vi "Discrete Transfer Function (DBL).vi"(2 "initialize":bool, 3 "transfer function":cluster{"numerator":dbl[], "denominator":dbl[]} {"denominator" format="%.2f"; "numerator" format="%.2f"}, 5 "input point":dbl format="%.2f") -> (1 "output point":dbl format="%.2f")   [LabVIEW 2020, in "NI_AdvCtrl_discrete linear.lvlib"]
doc: "LabVIEW no longer supports this VI. You can obtain similar functionality by installing the LabVIEW Simulation Module.\n\nCalculates the new output point, where the transfer function and the input point are given. The transfer function is described by two polynomials, numerator and denominator."
uses:
  <vilib>/addons/control/advanced/NI_AdvCtrl_discrete linear.lvlib
  <vilib>/addons/control/advanced/NI_AdvCtrl_continuous linear.lvlib
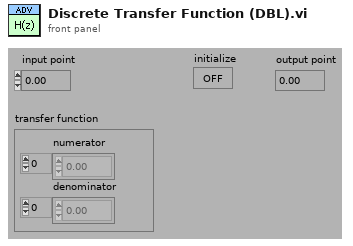
[diagram p1: front panel]
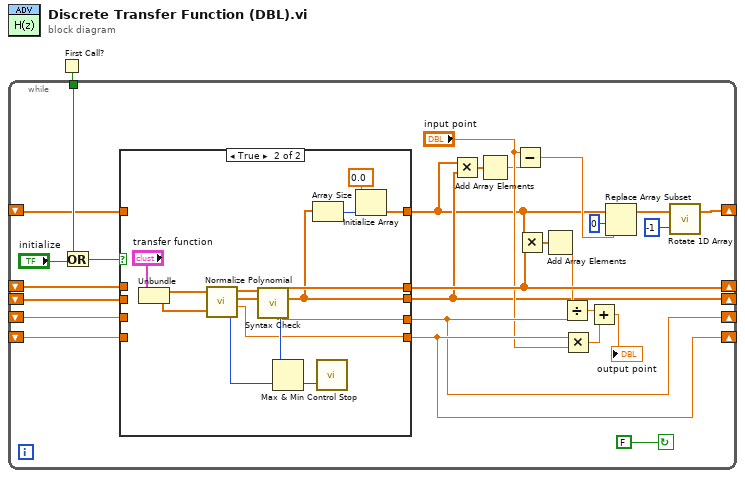
[diagram p0: block diagram]
diagram:
  n1 = First Call?() -> (First Call?: T/F=w1:bool)
  n2 = while {
    shift-left: _ -> [w13]
    shift-right: [w3] -> _
    tunnel: w1 -> [w17]
    shift-left: _ -> [w23]
    shift-right: [w22] -> _
    shift-left: _ -> [w24]
    shift-right: [w21] -> _
    shift-left: _ -> [w25]
    shift-right: [w7] -> _
    shift-left: _ -> [w26]
    shift-right: [w12] -> _
    stop <- FALSE continue-if-true
    n3 = Or(x=w17, y="initialize") -> (x .or. y?=w16:bool)
    n4 = case shown="True" w16 {
      tunnel: [w30 w44] -> w22
      tunnel: [w31 w43] -> w21
      tunnel: [w33 w42] -> w12
      tunnel: [w32 w39] -> w7
      tunnel: w26 -> [w33 _]
      tunnel: w25 -> [w32 _]
      tunnel: w24 -> [w31 _]
      tunnel: w23 -> [w30 _]
      tunnel: [w29 w38] -> w6
      tunnel: w13 -> [w29 _]
      frame False {
      }
      frame True {
        n5 = Unbundle("transfer function") -> ("numerator"=w37:dbl[], "denominator"=w36:dbl[])
        n6 = call <vilib>:"Normalize Polynomial.vi"("Numerator"=w37, "Denominator"=w36) -> ("Numerator new"=w45:dbl[], "Denominator new"=w46:dbl[], "additive constant"=w44:dbl, "error"=w47:i32)
        n7 = call <vilib>:"Syntax Check.vi"("Denominator"=w46, "Numerator"=w45) -> ("error"=w48:i32, "gain"=w43:dbl, "Denominator new"=w39:dbl[], "Numerator new"=w42:dbl[])  [unwired: 1 out]
        n8 = Max & Min(x=w48, y=w47) -> (min(x,y)=w35:i32)  [unwired: 1 out]
        n9 = Array Size(array=w39) -> (size(s)=w40:i32)
        n10 = call <vilib>:"Control Stop.vi"("error"=w35) -> ()  [unwired: 2 out]
        n11 = Initialize Array(0.0, w40) -> (w38:dbl[])
      }
    }
    n12 = Multiply(x=w6, y=w7) -> (x*y=w8:dbl[])
    n13 = Add Array Elements(numeric array=w8) -> (sum=w5:dbl)
    n14 = Subtract(x="input point", y=w5) -> (x-y=w15:dbl)
    n15 = Multiply(x=w6, y=w12) -> (x*y=w11:dbl[])
    n16 = Add Array Elements(numeric array=w11) -> (sum=w10:dbl)
    n17 = Divide(x=w10, y=w21) -> (x/y=w27:dbl)
    n18 = Multiply(x=w22, y="input point") -> (x*y=w28:dbl)
    n19 = Add(x=w27, y=w28) -> (x+y=→"output point":dbl)
    n20 = Replace Array Subset(array=w6, new element=w15, index=0 ("Index")) -> (w2:dbl[])
    n21 = call <vilib>:"Rotate 1D Array.vi"("n"=-1, "array"=w2) -> ("array (last n elements first)"=w3:dbl[])  [unwired: 1 out]
  }
